vi "Main.vi"() -> ()   [LabVIEW 2021]
uses:
  <vilib>/myRIO/Express VI/Onboard IO/Encoder/Encoder Express VI.xnode
  <vilib>/myRIO/Instrument Drivers/Onboard IO/Encoder/vis/Read.vi
  <vilib>/myRIO/Instrument Drivers/Onboard IO/Encoder/Encoder.lvlib
  <vilib>/myRIO/Common/Instrument Driver Framework/myRIO v1.0/Encoder/typedefs/Encoder Signal Mode.ctl
  <vilib>/myRIO/Common/Instrument Driver Framework/myRIO v1.0/Encoder/typedefs/Encoder Channels Enum.ctl
  <vilib>/myRIO/Common/Instrument Driver Framework/Utilities/typedefs/Generic FPGA Reference.ctl
  <vilib>/myRIO/Common/Instrument Driver Framework/Utilities/typedefs/myRIO v1.0 Reference.ctl
  <vilib>/myRIO/Common/Instrument Driver Framework/Utilities/typedefs/Hardware Version Enum.ctl
  <vilib>/myRIO/Common/Instrument Driver Framework/Utilities/typedefs/myRIO Generic Hardware Reference.ctl
  <vilib>/myRIO/Instrument Drivers/Onboard IO/Encoder/typedefs/Encoder Reference.ctl
  <vilib>/myRIO/Instrument Drivers/Onboard IO/Encoder/vis/myRIO Encoder Open.xnode
  <vilib>/myRIO/Common/Instrument Driver Framework/Utilities/vis/Is FPGA Ref Available.vi
  <vilib>/myRIO/Common/Instrument Driver Framework/myRIO v1.0/Encoder/typedefs/Encoder Configuration v1.0.ctl
  <vilib>/userDefined/High Color/nirio_resource_hc.ctl
  <vilib>/Simulation/Scripting/Companion Diagram/SimConfigNode/SimDog.xnode
  <vilib>/Simulation/Implementation/Shared/SIMSCR Execution Mode.ctl
  <vilib>/Simulation/Scripting/Companion Diagram/SimConfigNode/_simSolvers.ctl
  <vilib>/Simulation/Scripting/Companion Diagram/SimConfigNode/SimParams.ctl
  <vilib>/Platform/TimedLoop/XDataNode/XDataNode.xnode
  <vilib>/Platform/TimedLoop/XDataNode/nitl_modes.ctl
  <vilib>/Platform/TimedLoop/XDataNode/XDNodeRunTimeDep.lvlib
  <vilib>/Platform/TimedLoop/XDataNode/wakeup.ctl
  <vilib>/Platform/TimedLoop/XDataNode/timing_clust.ctl
  <vilib>/Simulation/Implementation/XNodeFramework/SimXNode/SimX.xnode
  <vilib>/Simulation/DataSources/Implementation/NILVSim Pulse Generator.llb/SIM Pulse Generator (scalar).vi
  <vilib>/Simulation/SignalDisplay/Implementation/NILVSim Time Waveform.llb/SIM Time Waveform (vector).vi
  <vilib>/Simulation/SignalArithmetic/Implementation/NILVSim Gain.llb/SIM Gain (scalar).vi
  <vilib>/Simulation/ContinuousLinear/Implementation/NILVSim Transfer Function Direct.llb/SIM Transfer Function Direct (SISO).vi
  <vilib>/Simulation/Utility/Implementation/SIM Halt.vi
  <vilib>/Simulation/DataSources/Implementation/NILVSim Step.llb/SIM Step (scalar).vi
  <vilib>/Simulation/DataSources/Implementation/NILVSim Sine Wave.llb/SIM Sine Wave (scalar).vi
  <vilib>/Simulation/ContinuousLinear/Implementation/NILVSim Integrator new.llb/SIM Integrator (scalar).vi
  <vilib>/myRIO/Common/Instrument Driver Framework/myRIO v1.0/Encoder/vis/myRIO v1.1 Open Encoder.vi
  <vilib>/myRIO/Common/Instrument Driver Framework/myRIO v1.0/Encoder/vis/myRIO v1.0 Configure Encoder.vi
  <vilib>/myRIO/Express VI/Onboard IO/PWM/PWM Express VI.xnode
  <vilib>/myRIO/Instrument Drivers/Onboard IO/PWM/vis/Set Duty Cycle and Frequency.vi
  <vilib>/myRIO/Instrument Drivers/Onboard IO/PWM/PWM.lvlib
  <vilib>/myRIO/Instrument Drivers/Onboard IO/PWM/typedefs/PWM Configuration.ctl
  <vilib>/myRIO/Common/Instrument Driver Framework/myRIO v1.0/PWM/typedefs/PWM Channels Enum.ctl
  <vilib>/myRIO/Instrument Drivers/Onboard IO/PWM/typedefs/PWM Reference.ctl
  <vilib>/myRIO/Instrument Drivers/Onboard IO/PWM/vis/myRIO PWM Open.xnode
  <vilib>/myRIO/Common/Instrument Driver Framework/myRIO v1.0/PWM/vis/myRIO v1.1 Open PWM.vi
  <vilib>/Simulation/Implementation/Shared/SIM Bundle Sim Info.vi
  <vilib>/Simulation/Implementation/Shared/SIM Unbundle Sim Info.vi
  <vilib>/Simulation/Implementation/Shared/NILVSim_FinalizeModel.vi
  <vilib>/Simulation/Implementation/Shared/NILVSim_GetModelError.vi
  <vilib>/Simulation/Implementation/Shared/NILVSim_Initialize.vi
  <vilib>/Simulation/Implementation/Shared/NILVSim_FinishedLate.vi
  <vilib>/Simulation/Utility/Implementation/NILVSim Get Time and IsAcceptedStep.vi
  <vilib>/Simulation/Implementation/Shared/NILVSim_Manager.vi
  <vilib>/Simulation/Implementation/Shared/NI_SIM_Implementation.lvlib
  <vilib>/Simulation/Implementation/Shared/NILVSIM_BeginStep.vi
  <vilib>/Simulation/Param Hierarchy/Typedefs/SIMPH Param Control Actions.ctl
  <vilib>/Simulation/Implementation/Shared/NILVSim_ParamChanged.vi
  <vilib>/Utility/error.llb/Clear Errors.vi
  <vilib>/Simulation/Implementation/Shared/SIMSH Read Queue.vi
  <vilib>/Simulation/Utility/Implementation/NILVSim Memory.llb/NILVSim Memory (core).vi
  <vilib>/Simulation/ContinuousLinear/Implementation/NILVSim Integrator new.llb/SIM Integrator distributor (scalar).vi
  <vilib>/Simulation/ContinuousLinear/Implementation/NILVSim Integrator new.llb/SIM Integrator collector (scalar).vi
  <vilib>/Simulation/Implementation/Shared/SIM limit type.ctl
  <vilib>/myRIO/Common/Instrument Driver Framework/myRIO v1.0/Encoder/typedefs/Encoder Count Direction Enum.ctl
panel:
  in  "STOP":bool
  in  "Tab Control":T1(tab)
  out "Counter Value":i32
  out "Counter Direction":enum16{"Counting Up", "Counting Down"}(ring)
  in  "Reset Counter":bool
  in  "Step Collect Data":bool
  in  "Stop Step Controller":bool
  out "Step Voltage and Resultant Velocity":waveform(dbl)[](graph)
  in  "Step Final Time (s)":dbl=5.0 min=0.0 max=30.0 step=0.1
  in  "Step Voltage (V)":dbl=2.0 min=-20.0 max=20.0 step=0.1
  in  "Encoder Step Count":dbl format="%#_13g"
  in  "Sine Freq. (Hz)":dbl=2.0 min=0.0 max=100.0 step=0.1
  in  "Sine Collect Data":bool
  in  "Stop Sine Controller":bool
  out "Sine Voltage and Resultant Velocity":waveform(dbl)[](graph)
  in  "Sine Final Time (s)":dbl=5.0 min=0.0 max=30.0 step=0.1
  in  "Sine Voltage (V)":dbl=2.0 min=-20.0 max=20.0 step=0.1
  in  "Encoder step count":dbl format="%#_13g"
  out "Pulse Desired and Actual Position":waveform(dbl)[](graph)
  in  "Pulse Final Time (s)":dbl=5.0 min=0.0 max=30.0 step=0.1
  in  "Pulse Period (s)":dbl=2.0 min=0.0 max=30.0 step=0.1
  in  "Pulse Desired\nPosition (Radians)":dbl=1.0 min=-6.3 max=6.3 step=0.1
  in  "Pulse Kp":dbl min=0.0 max=1000.0 step=0.01
  in  "Pulse Kd":dbl min=0.0 max=1000.0 step=0.01
  in  "Pulse Ki":dbl min=0.0 max=1000.0 step=0.01
  in  "Stop Pulse Controller":bool
  in  "Pulse Collect Data":bool
  in  "Encoder step count":dbl format="%#_13g"
  in  "Driver gauge":dbl(knob)=175.96184714110825 scale=0.0..360.0
  out "Encoder gauge":dbl(knob)=175.96184714110825 scale=0.0..360.0
  out "Desired and Actual Position":waveform(dbl)[](graph)
  in  "Ki":dbl min=0.0 max=1000.0 step=0.01
  in  "Kd":dbl min=0.0 max=1000.0 step=0.01
  in  "Kp":dbl min=0.0 max=1000.0 step=0.01
  # "Bug Note:\nFirst run of each graph after starting VI\nproduces incorrect readings for the\nfirst second.  Second and subsequent\nruns are unaffected."
  # "Bug Note:\nFirst run of each graph after starting VI\nproduces incorrect readings for the\nfirst second.  Second and subsequent\nruns are unaffected."
  # "Bug Note:\nFirst run of each graph after starting VI\nproduces incorrect readings for the\nfirst second.  Second and subsequent\nruns are unaffected."
  # "Red = control input for position\nOrange = what position the encoder is seeing"
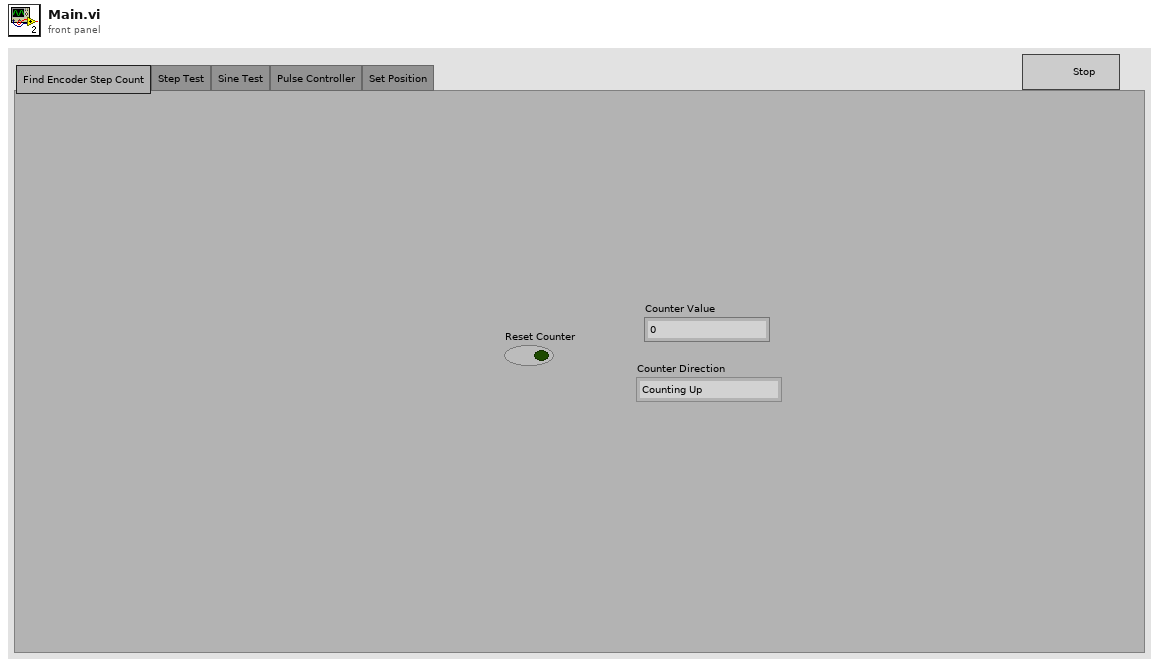
[diagram p1: front panel]
types:
  T1 = enum32{"Find Encoder Step Count", "Step Test", "Sine Test", "Pulse Controller", "Set Position"}
  T2 = typedef "XDNodeRunTimeDep.lvlib/timing_clust.ctl" = cluster{"Expected End [f-1]":u64, "Actual End [f-1]":u64, "Finished Late? [f-1]":bool, "Expected End [i-1]":u64, "Actual End [i-1]":u64, "Finished Late? [i-1]":bool, "Expected Start [i]":u64, "Actual Start [i]":u64, "Expected Start [f]":u64, "Actual Start [f]":u64, "Source Name":string, "Structure Name":string, "Period":i64, "Deadline":i64, "Offset":i64, "Start":i64, "Priority":i32, "Timeout":i32, "Mode":T3, "Wakeup Reason":T4, "Error":errorcluster, "Source Type":string, "Secondary Source Type":string, "Global End Time":u64, "Global Start Time":u64, "Frame Duration":u64, "Iteration Duration":u64, "Assigned CPU":i32, "I/O Scan Engine Mode":u32}
  T3 = typedef "XDNodeRunTimeDep.lvlib/nitl_modes.ctl" = enum32{"No Change", "Process missed periods, maintain original phase", "Discard missed periods, maintain original phase", "Process missed periods, ignore original phase", "Discard missed periods, ignore original phase"}
  T4 = typedef "XDNodeRunTimeDep.lvlib/wakeup.ctl" = enum32{"Normal", "Aborted", "Asynchronous wakeup", "Timing source error", "Timed loop error", "Timeout"}
  T5 = typedef "Encoder.lvlib/Encoder Reference.ctl" = cluster{"myRIO Reference":T6, "Encoder Channels Enum":T10}
  T6 = typedef "myRIO Generic Hardware Reference.ctl" = cluster{"myRIO Model":T7, "myRIO Hardware Reference":T8}
  T7 = typedef "Hardware Version Enum.ctl" = enum16{"Unknown", "myRIO-1900", "myRIO-1950", "roboRIO", "NI ELVIS RIO CM", "ELVIS III"}
  T8 = typedef "myRIO v1.0 Reference.ctl" = cluster{"Generic FPGA Reference":T9, "Allow multiple opens":bool}
  T9 = typedef "Generic FPGA Reference.ctl" = refnum<k20>
  T10 = typedef "Encoder Channels Enum.ctl" = enum16{"Not Connected", "C/ENC0", "C/ENC1", "A/ENC", "A/ENC0", "A/ENC1", "A/ENC2", "A/ENC3", "A/ENC4", "A/ENC5", "A/ENC6", "A/ENC7", "A/ENC8", "A/ENC9", "B/ENC", "B/ENC0", "B/ENC1", "B/ENC2", "B/ENC3", "B/ENC4", "B/ENC5", "B/ENC6", "B/ENC7", "B/ENC8", "B/ENC9", "DIO/ENC0", "DIO/ENC1", "DIO/ENC2", "DIO/ENC3", "DIO/ENC4"}
  T11 = typedef "Encoder Signal Mode.ctl" = enum16{"Quadrature phase signal", "Step and direction signal"}
  T12 = typedef "nirio_resource_hc.ctl" = tag
  T13 = typedef "PWM.lvlib/PWM Reference.ctl" = cluster{"myRIO Reference":T6, "PWM Channels Enum":T14, "PWM Configuration":T15}
  T14 = typedef "PWM Channels Enum.ctl" = enum16{"Not Connected", "C/PWM0", "C/PWM1", "A/PWM0", "A/PWM1", "A/PWM2", "A/PWM3", "A/PWM4", "A/PWM5", "A/PWM6", "A/PWM7", "A/PWM8", "A/PWM9", "A/PWM10", "A/PWM11", "A/PWM12", "A/PWM13", "A/PWM14", "A/PWM15", "A/PWM16", "A/PWM17", "A/PWM18", "A/PWM19", "B/PWM0", "B/PWM1", "B/PWM2", "B/PWM3", "B/PWM4", "B/PWM5", "B/PWM6", "B/PWM7", "B/PWM8", "B/PWM9", "B/PWM10", "B/PWM11", "B/PWM12", "B/PWM13", "B/PWM14", "B/PWM15", "B/PWM16", "B/PWM17", "B/PWM18", "B/PWM19", "PWM/PWM0", "PWM/PWM1", "PWM/PWM2", "PWM/PWM3", "PWM/PWM4", "PWM/PWM5", "PWM/PWM6", "PWM/PWM7", "PWM/PWM8", "PWM/PWM9"}
  T15 = typedef "PWM.lvlib/PWM Configuration.ctl" = cluster{"Frequency":dbl, "Duty Cycle":dbl}
  T16 = typedef "SIMSCR Execution Mode.ctl" = enum16{"Simulate to Completion", "Single Time-Step Simulation (Fixed Step Only)"}
  T17 = typedef "SIMPH Param Control Actions.ctl" = enum16{"get params", "set params"}
  T18 = typedef "SimParams.ctl" = cluster{"Initial Time (s)":dbl, "Final Time (s)":dbl, "Step Size (s)":dbl, "ODE Solver":T19, "Minimum Step Size (s)":dbl, "Maximum Step Size (s)":dbl, "Relative Tolerance":dbl, "Absolute Tolerance":dbl, "Software Timing":bool, "Initial Step Size (s)":dbl, "Automatic Fixed Step Size?":bool, "Automatic Discrete Step Size?":bool, "Discrete Step Size (s)":dbl, "Calculate using Time Step":bool, "Solver Wired?":bool, "Prev.Frm.Expected End":u64, "Prev.Frm.Actual End":u64, "Prev.Frm.Finished Late?":bool, "Prev.Iter.Expected End":u64, "Prev.Iter.Actual End":u64, "Prev.Iter.Finished Late?":bool, "Expected Iteration Start":u64, "Actual Iteration Start":u64, "Expected Frame Start":u64, "Actual Frame Start":u64, "Source Name":string, "Name":string, "Period":i64, "Deadline":i64, "Offset":i64, "Start":i64, "Priority":i32, "Timeout":i32, "Processor":i32, "Mode":enum32{"No Change", "Process missed periods, maintain original phase", "Discard missed periods, maintain original phase", "Process missed periods, ignore original phase", "Discard missed periods, ignore original phase"}, "Wakeup reason":enum32{"Normal", "Aborted", "Asynchronous wakeup", "Timing source error", "Timed loop error", "Timeout"}, "Error":errorcluster, "Source Type":string, "Secondary Source Type":string, "Global End Time":u64, "Global Start Time":u64, "Full Solver Reset":bool, "Execution Mode":T16, "Nan/Inf Check":bool, "Custom Solver Library":string, "Solver Is Variable":bool, "custom solver name":string, "Signal Collection Decimation":u32}
  T19 = typedef "_simSolvers.ctl" = enum16{"Runge-Kutta 1 (Euler)", "Runge-Kutta 2", "Runge-Kutta 3", "Runge-Kutta 4", "Runge-Kutta 23 (variable)", "Runge-Kutta 45 (variable)", "BDF (variable)", "Adams-Moulton (variable)", "Rosenbrock (variable)", "Discrete States Only", "SDIRK 4 (variable)", "Radau 5 (variable)", "Radau 9 (variable)", "Radau 13 (variable)", "Radau [Variable Order] (variable)", "Gear's Method (variable)", "Linearizer", "State Query", "Trim Eval", "Custom Solver"}
  T20 = typedef "SIM limit type.ctl" = enum16{"upper", "lower", "both", "none"}
  T21 = typedef "Encoder Count Direction Enum.ctl" = enum16{"Counting Up", "Counting Down"}
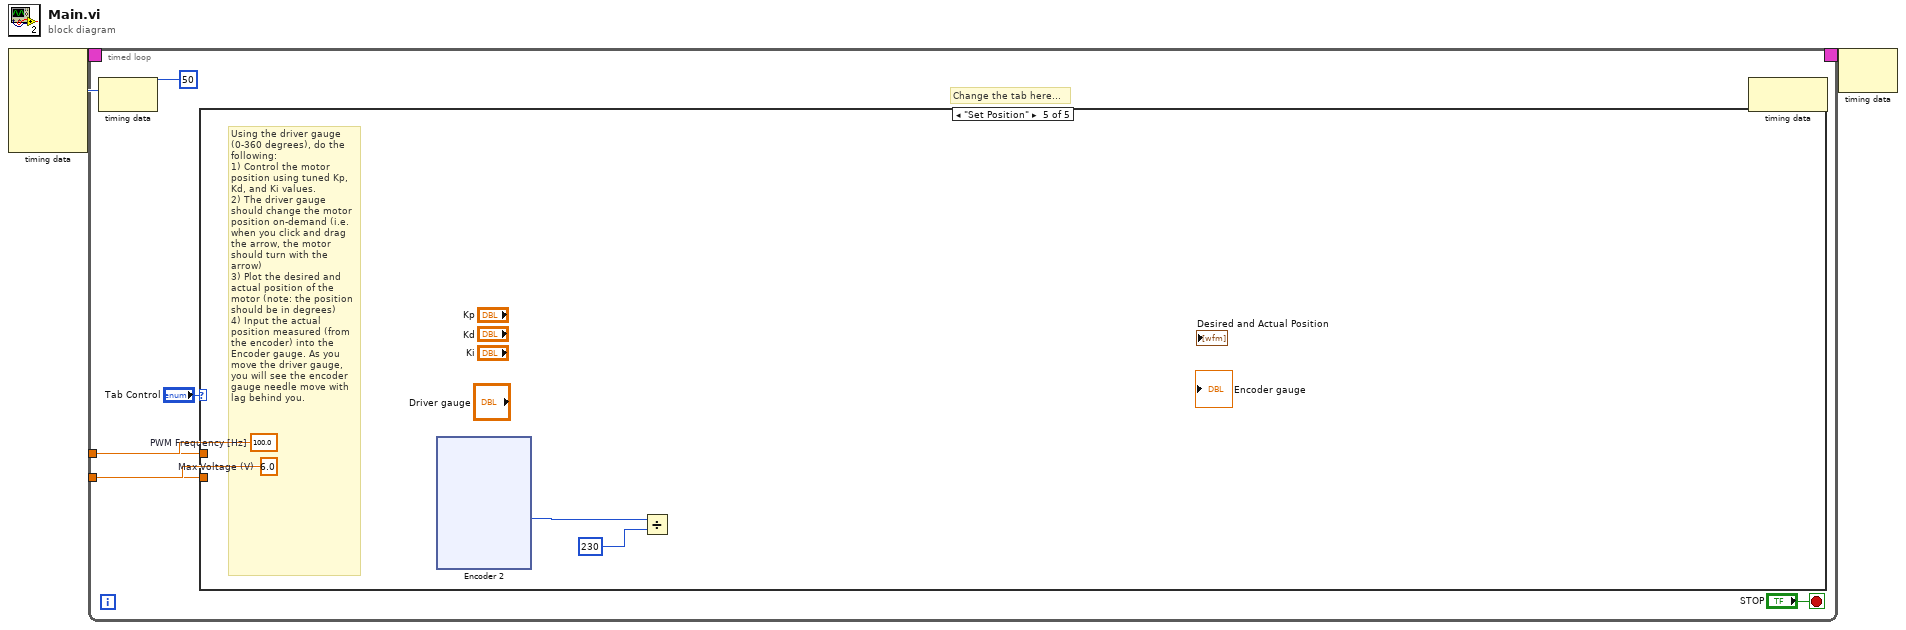
[diagram p0: block diagram]
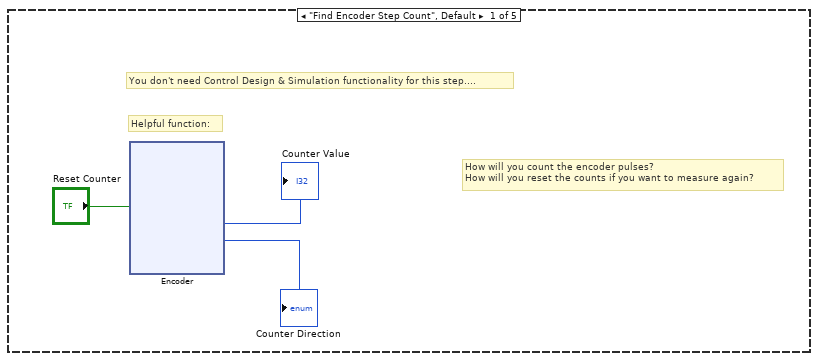
[diagram p2: hidden frame]
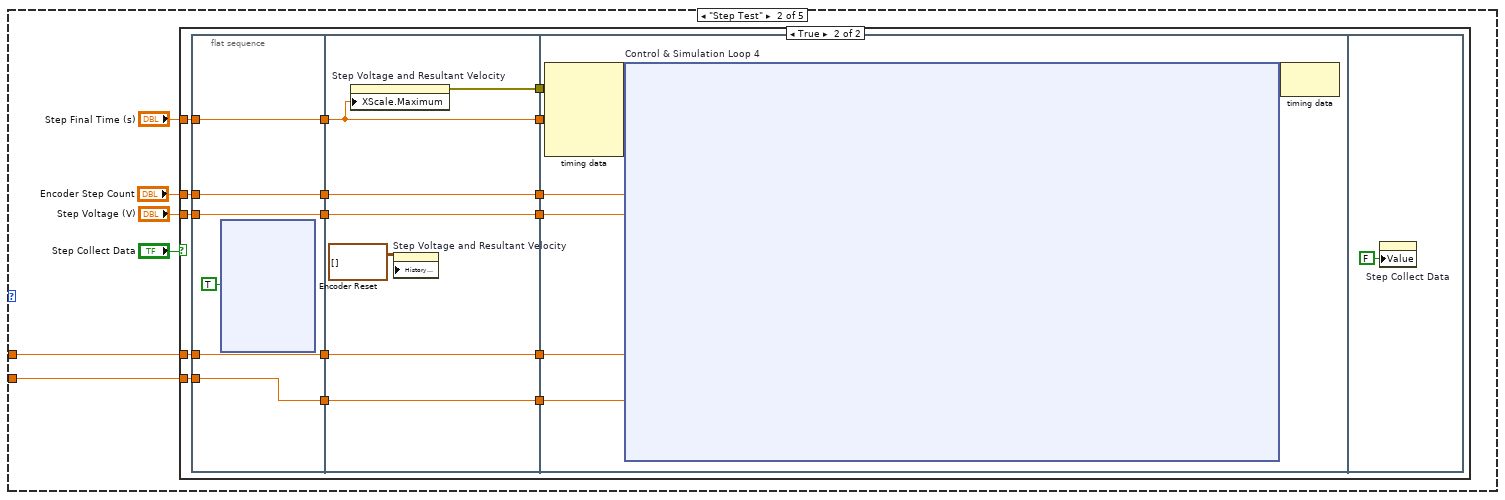
[diagram p3: hidden frame]
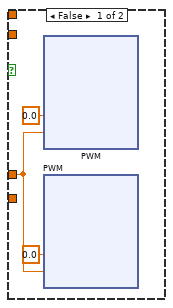
[diagram p4: hidden frame]
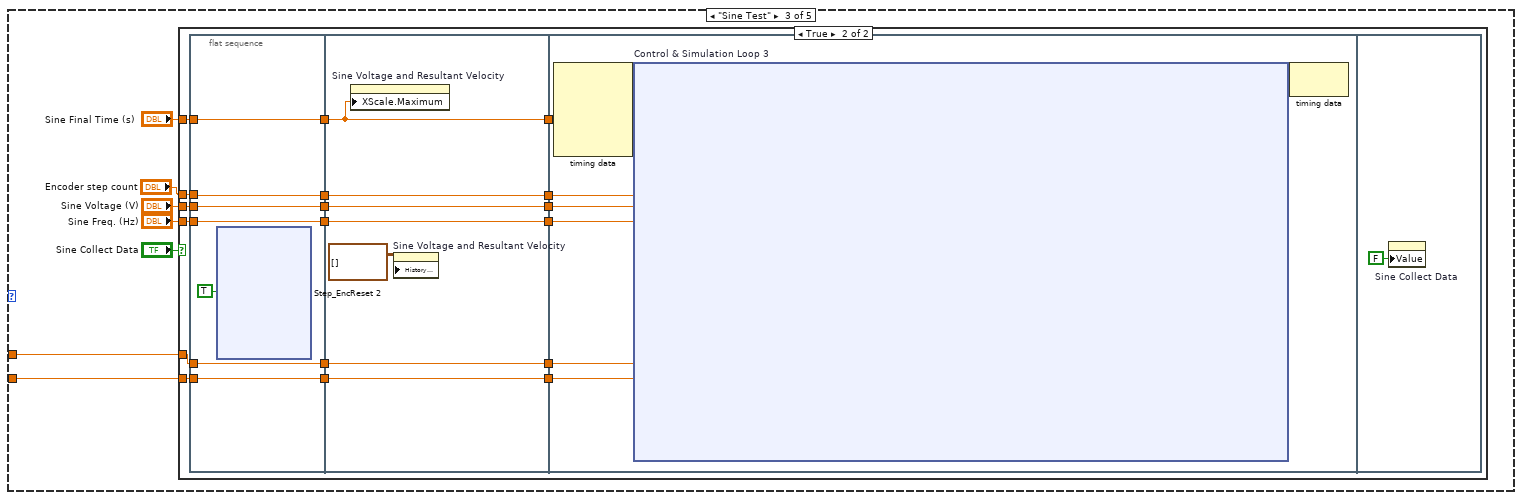
[diagram p5: hidden frame]
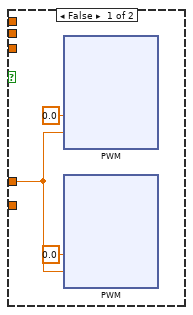
[diagram p6: hidden frame]
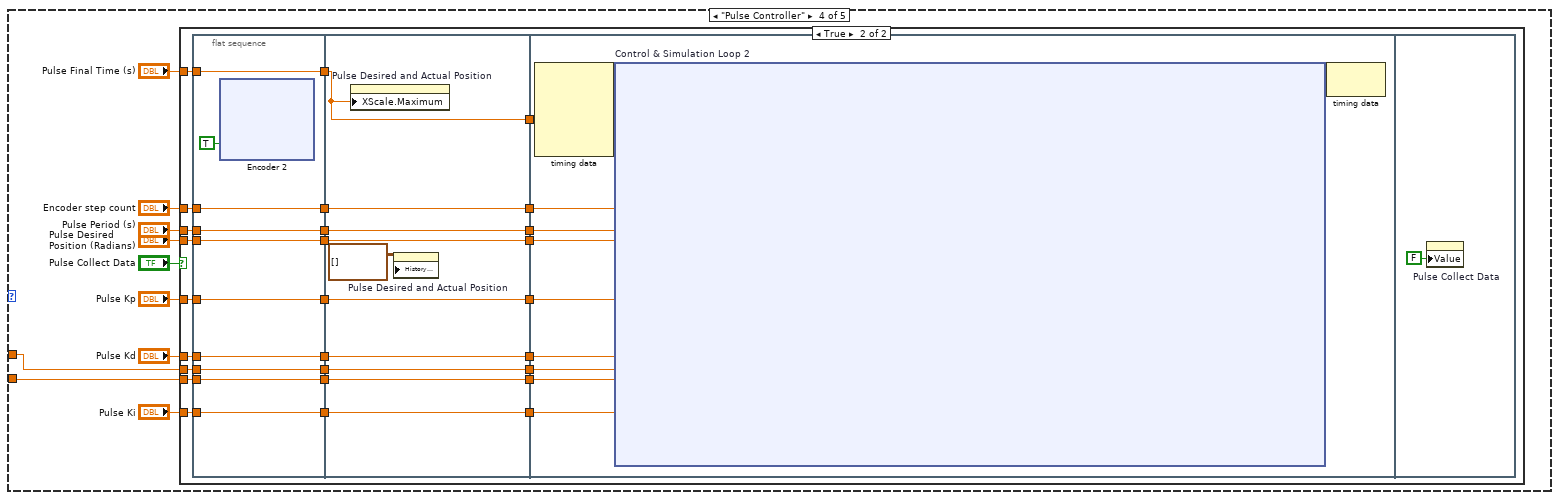
[diagram p7: hidden frame]
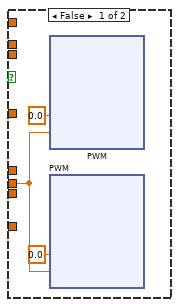
[diagram p8: hidden frame]
diagram:
  w1 = 6.0  # Max Voltage (V)
  w2 = 100.0  # PWM Frequency [Hz]
  n1 = node-c288(i64 50 ("Period")) -> (w5:T2)  [unwired: 4 in]
  n2 = timed-loop {
    timing: w5 -> [_]
    timing-out: [_] -> w4
    tunnel: w2 -> [w7]
    tunnel: w1 -> [w6]
    stop <- "STOP" stop-if-true
    # "Change the tab here..."
    n3 = node-c288() -> ()  [unwired: 1 in, 1 out]
    n4 = case shown="\"Set Position\"" "Tab Control" {
      tunnel: w7 -> [_ w61 w880 w1713 _]
      tunnel: w6 -> [_ w60 w879 w1714 _]
      frame "Find Encoder Step Count", Default {
        # "How will you count the encoder pulses?\nHow will you reset the counts if you want to measure again?"
        # "You don't need Control Design & Simulation functionality for this step...."
        # "Helpful function:"
        n5 = xnode "Encoder"("Reset Counter"="Reset Counter") -> ("Counter Value"=→"Counter Value":i32, "Counter Direction"=→"Counter Direction":T21)  [unwired: 1 in, 2 out]
      }
      frame "Step Test" {
        n6 = case shown="True" "Step Collect Data" {
          tunnel: "Step Final Time (s)" -> [_ w153]
          tunnel: "Step Voltage (V)" -> [_ w152]
          tunnel: w61 -> [w66 w144]
          tunnel: w60 -> [_ w141]
          tunnel: "Encoder Step Count" -> [_ w138]
          frame False {
            n7 = xnode ("PWM")("Duty Cycle"=0.0 ("A/AO0"), "Frequency [Hz]"=w66) -> ()  [unwired: 1 in, 1 out]
            n8 = xnode ("PWM")("Duty Cycle"=0.0, "Frequency [Hz]"=w66) -> ()  [unwired: 1 in, 1 out]
          }
          frame True {
            n9 = flat-sequence {
              tunnel: w152 -> [w158]
              tunnel: w153 -> [w159]
              tunnel: [w159] -> w148
              tunnel: [w158] -> w147
              tunnel: [w156] -> w145
              tunnel: w144 -> [w156]
              tunnel: [w155] -> w142
              tunnel: w141 -> [w155]
              tunnel: [w154] -> w140
              tunnel: w138 -> [w154]
              tunnel: [w210] -> w151
              tunnel: [w212] -> w150
              tunnel: [w209] -> w149
              tunnel: w148 -> [w210]
              tunnel: w147 -> [w212]
              tunnel: [w208] -> w146
              tunnel: w145 -> [w208]
              tunnel: [w207] -> w143
              tunnel: w142 -> [w207]
              tunnel: w140 -> [w206]
              tunnel: [w206] -> w139
              tunnel: w151 -> [w218]
              tunnel: w150 -> [w217]
              tunnel: w149 -> [w216]
              tunnel: w146 -> [w215]
              tunnel: w143 -> [w214]
              tunnel: w139 -> [w213]
              frame #0 {
                n10 = xnode "Encoder Reset"("Reset Counter"=TRUE) -> ()  [unwired: 1 in, 4 out]
              }
              frame #1 {
                n11 = property on="Step Voltage and Resultant Velocity" class="WFChart (strict)"("XScale.Maximum"=w210) -> (error out=w209:errorcluster)  [unwired: 2 in, 1 out]
                n12 = property on="Step Voltage and Resultant Velocity" class="WFChart (strict)"("History Data"=waveform(dbl)[][] []) -> ()  [unwired: 2 in, 2 out]
              }
              frame #2 {
                n13 = node-c288(w216, w218) -> (w220:variant)  [unwired: 3 in]
                n14 = node-c254 "Control & Simulation Loop 4"(w220, w217, w215, w214, w213) -> (w219:variant)
                n15 = node-c288(w219) -> ()  [unwired: 1 out]
              }
              frame #3 {
                n16 = property on="Step Collect Data" class="Bool (strict)"("Value"=FALSE ("Collect Data")) -> ()  [unwired: 2 in, 2 out]
              }
            }
          }
        }
      }
      frame "Sine Test" {
        n17 = case shown="True" "Sine Collect Data" {
          tunnel: "Sine Final Time (s)" -> [_ w975]
          tunnel: "Sine Voltage (V)" -> [_ w974]
          tunnel: "Sine Freq. (Hz)" -> [_ w971]
          tunnel: w880 -> [w885 w964]
          tunnel: w879 -> [_ w963]
          tunnel: "Encoder step count" -> [_ w958]
          frame False {
            n18 = xnode ("PWM")("Duty Cycle"=0.0 ("A/AO0"), "Frequency [Hz]"=w885) -> ()  [unwired: 1 in, 1 out]
            n19 = xnode ("PWM")("Duty Cycle"=0.0, "Frequency [Hz]"=w885) -> ()  [unwired: 1 in, 1 out]
          }
          frame True {
            n20 = flat-sequence {
              tunnel: w971 -> [w980]
              tunnel: w974 -> [w981]
              tunnel: w975 -> [w982]
              tunnel: [w982] -> w969
              tunnel: [w981] -> w968
              tunnel: [w980] -> w967
              tunnel: [w979] -> w965
              tunnel: w964 -> [w979]
              tunnel: w963 -> [w977]
              tunnel: [w977] -> w962
              tunnel: w958 -> [w976]
              tunnel: [w976] -> w960
              tunnel: [w1033] -> w973
              tunnel: [w1035] -> w972
              tunnel: [w1032] -> w970
              tunnel: w969 -> [w1033]
              tunnel: w968 -> [w1035]
              tunnel: w967 -> [w1032]
              tunnel: [w1031] -> w966
              tunnel: w965 -> [w1031]
              tunnel: w962 -> [w1030]
              tunnel: [w1030] -> w961
              tunnel: w960 -> [w1029]
              tunnel: [w1029] -> w959
              tunnel: w973 -> [w1041]
              tunnel: w972 -> [w1040]
              tunnel: w970 -> [w1039]
              tunnel: w966 -> [w1038]
              tunnel: w961 -> [w1037]
              tunnel: w959 -> [w1036]
              frame #0 {
                n21 = xnode "Step_EncReset 2"("Reset Counter"=TRUE) -> ()  [unwired: 1 in, 4 out]
              }
              frame #1 {
                n22 = property on="Sine Voltage and Resultant Velocity" class="WFChart (strict)"("XScale.Maximum"=w1033) -> ()  [unwired: 2 in, 2 out]
                n23 = property on="Sine Voltage and Resultant Velocity" class="WFChart (strict)"("History Data"=waveform(dbl)[][] []) -> ()  [unwired: 2 in, 2 out]
              }
              frame #2 {
                n24 = node-c288(w1041) -> (w1043:variant)  [unwired: 4 in]
                n25 = node-c254 "Control & Simulation Loop 3"(w1043, w1040, w1039, w1038, w1037, w1036) -> (w1042:variant)
                n26 = node-c288(w1042) -> ()  [unwired: 1 out]
              }
              frame #3 {
                n27 = property on="Sine Collect Data" class="Bool (strict)"("Value"=FALSE ("Collect Data")) -> ()  [unwired: 2 in, 2 out]
              }
            }
          }
        }
      }
      frame "Pulse Controller" {
        n28 = case shown="True" "Pulse Collect Data" {
          tunnel: "Pulse Final Time (s)" -> [_ w1821]
          tunnel: "Pulse Period (s)" -> [_ w1820]
          tunnel: "Pulse Desired\nPosition (Radians)" -> [_ w1819]
          tunnel: "Pulse Kd" -> [_ w1818]
          tunnel: "Pulse Kp" -> [_ w1817]
          tunnel: "Pulse Ki" -> [_ w1816]
          tunnel: w1714 -> [_ w1801]
          tunnel: w1713 -> [w1722 w1798]
          tunnel: "Encoder step count" -> [_ w1795]
          frame False {
            n29 = xnode ("PWM")("Duty Cycle"=0.0 ("A/AO0"), "Frequency [Hz]"=w1722) -> ()  [unwired: 1 in, 1 out]
            n30 = xnode ("PWM")("Duty Cycle"=0.0, "Frequency [Hz]"=w1722) -> ()  [unwired: 1 in, 1 out]
          }
          frame True {
            n31 = flat-sequence {
              tunnel: w1816 -> [w1826]
              tunnel: w1817 -> [w1827]
              tunnel: w1818 -> [w1828]
              tunnel: w1819 -> [w1829]
              tunnel: w1820 -> [w1830]
              tunnel: w1821 -> [w1831]
              tunnel: [w1831] -> w1809
              tunnel: [w1830] -> w1808
              tunnel: [w1829] -> w1807
              tunnel: [w1828] -> w1806
              tunnel: [w1827] -> w1805
              tunnel: [w1826] -> w1804
              tunnel: [w1825] -> w1802
              tunnel: w1801 -> [w1825]
              tunnel: [w1824] -> w1799
              tunnel: w1798 -> [w1824]
              tunnel: w1795 -> [w1822]
              tunnel: [w1822] -> w1797
              tunnel: [w1881] -> w1815
              tunnel: [w1887] -> w1814
              tunnel: [w1886] -> w1813
              tunnel: [w1885] -> w1812
              tunnel: [w1884] -> w1811
              tunnel: [w1883] -> w1810
              tunnel: w1809 -> [w1881]
              tunnel: w1808 -> [w1887]
              tunnel: w1807 -> [w1886]
              tunnel: w1806 -> [w1885]
              tunnel: w1805 -> [w1884]
              tunnel: w1804 -> [w1883]
              tunnel: [w1880] -> w1803
              tunnel: w1802 -> [w1880]
              tunnel: [w1879] -> w1800
              tunnel: w1799 -> [w1879]
              tunnel: w1797 -> [w1878]
              tunnel: [w1878] -> w1796
              tunnel: w1815 -> [w1896]
              tunnel: w1814 -> [w1895]
              tunnel: w1813 -> [w1894]
              tunnel: w1812 -> [w1893]
              tunnel: w1811 -> [w1892]
              tunnel: w1810 -> [w1891]
              tunnel: w1803 -> [w1890]
              tunnel: w1800 -> [w1889]
              tunnel: w1796 -> [w1888]
              frame #0 {
                n32 = xnode ("Encoder 2")("Reset Counter"=TRUE) -> ()  [unwired: 1 in, 4 out]
              }
              frame #1 {
                n33 = property on="Pulse Desired and Actual Position" class="WFChart (strict)"("XScale.Maximum"=w1881) -> ()  [unwired: 2 in, 2 out]
                n34 = property on="Pulse Desired and Actual Position" class="WFChart (strict)"("History Data"=waveform(dbl)[][] []) -> ()  [unwired: 2 in, 2 out]
              }
              frame #2 {
                n35 = node-c288(w1896) -> (w1898:variant)  [unwired: 4 in]
                n36 = node-c254 "Control & Simulation Loop 2"(w1898, w1895, w1894, w1893, w1892, w1891, w1890, w1889, w1888) -> (w1897:variant)
                n37 = node-c288(w1897) -> ()  [unwired: 1 out]
              }
              frame #3 {
                n38 = property on="Pulse Collect Data" class="Bool (strict)"("Value"=FALSE ("Collect Data")) -> ()  [unwired: 2 in, 2 out]
              }
            }
          }
        }
      }
      frame "Set Position" {
        # "Using the driver gauge (0-360 degrees), do the following:\n1) Control the motor position using tuned Kp, Kd, and Ki values.\n2) The driver gauge should change the motor position on-demand (i.e. when you click and drag the arrow, the motor should turn with the arrow)\n3) Plot the desired and actual position of the motor (note: the position should be in degrees)\n4) Input the actual position measured (from the encoder) into the Encoder gauge. As you move the driver gauge, you will see the encoder gauge needle move with lag behind you."
        n39 = xnode "Encoder 2"() -> ("Counter Value"=w2636:i32)  [unwired: 2 in, 3 out]
        n40 = Divide(x=w2636, y=230) -> ()  [unwired: 1 out]
      }
    }
    n41 = node-c288() -> ()  [unwired: 1 in, 1 out]
  }
  n42 = node-c288(w4) -> ()  [unwired: 1 out]
